vi "StopImageAcquisition.vi"(8 "error in (no error)":errorcluster, 11 "session in":T1) -> (0 "error out":errorcluster)   [LabVIEW 2017, in "IrAcquisition.lvlib"]
uses:
  <vilib>/addons/InsightCM/Devices/Shared/Ir/IrAcquisition/IrAcquisition.lvlib
  <vilib>/userdefined/High Color/IMAQdx.ctl
  <vilib>/vision/driver/NI_Vision_Acquisition_Software.lvlib
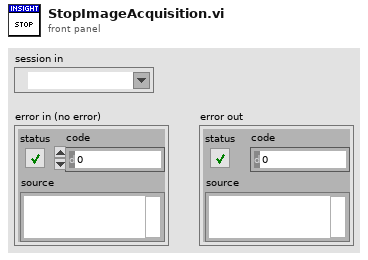
[diagram p1: front panel]
types:
  T1 = typedef "IMAQdx.ctl" = refnum<k21>
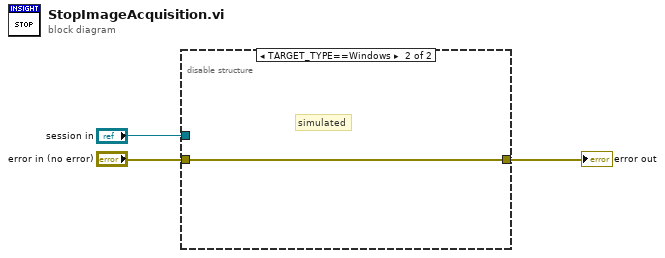
[diagram p0: block diagram]
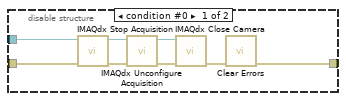
[diagram p2: hidden frame]
diagram:
  n1 = disable-structure shown="TARGET_TYPE==Windows" {
    disable-tunnel: [w11 w12] -> w3
    disable-tunnel: "session in" -> [w7 _]
    disable-tunnel: "error in (no error)" -> [w6 w12]
    frame condition #0 {
      n2 = call <vilib>:"IMAQdx Stop Acquisition.vi"("error in"=w6, "Session In"=w7) -> ("error out"=w8:errorcluster, "Session Out"=w5:T1)  [unwired: 8 out]
      n3 = call <vilib>:"IMAQdx Unconfigure Acquisition.vi"("error in"=w8, "Session In"=w5) -> ("error out"=w9:errorcluster, "Session Out"=w4:T1)  [unwired: 8 out]
      n4 = call <vilib>:"IMAQdx Close Camera.vi"("error in"=w9, "Session In"=w4) -> ("error out"=w10:errorcluster)  [unwired: 9 out]
      n5 = call <vilib>:"Clear Errors.vi"("error in (no error)"=w10) -> ("error out"=w11:errorcluster)  [unwired: 5 in, 1 out]
    }
    frame condition #1 (active) {
      # "simulated"
    }
  }
  "error out" <- w3
